vi "sendScript.vi"(8 "error in (no error)":errorcluster, 11 "K2602 in":refnum<class "K2602.lvclass">) -> (0 "error out":errorcluster, 3 "K2602 out":refnum<class "K2602.lvclass">)   [LabVIEW 2011, in "Hardware.lvlib" / "Channels.lvlib" / "K2602.lvclass"]
uses:
  K2602.lvclass
  K2602.lvclass/K2602.ctl
  <instrlib>/Keithley 2600 Series/Keithley 2600 Series.lvlib
panel:
  out "script":string
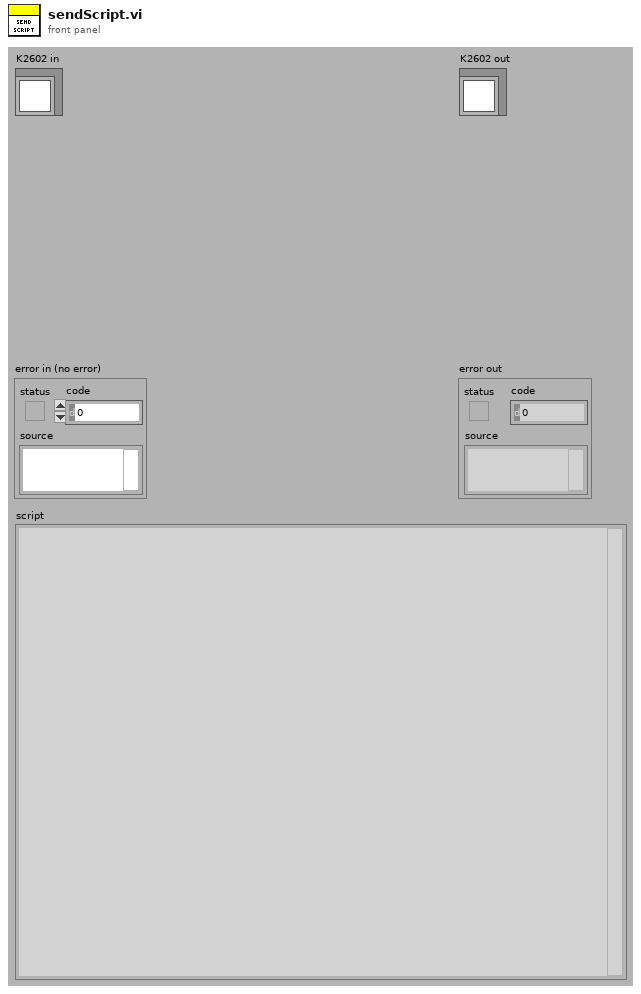
[diagram p1: front panel]
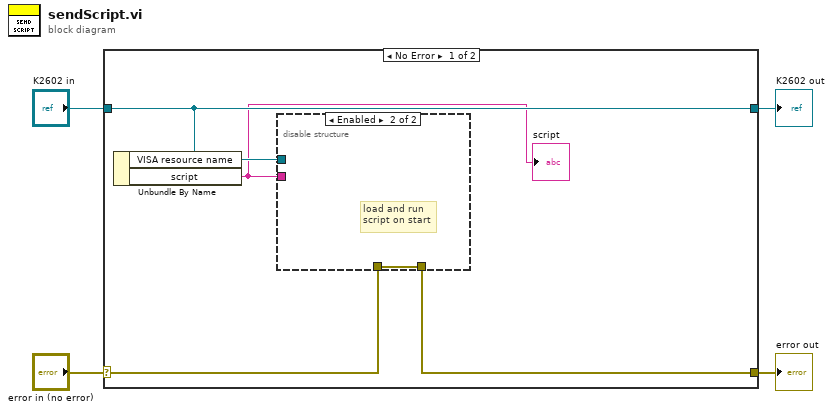
[diagram p0: block diagram]
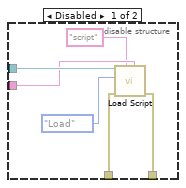
[diagram p2: hidden frame]
diagram:
  n1 = case shown="No Error" "error in (no error)" {
    selector: "error in (no error)" -> [w7 w18]
    tunnel: [w6 w18] -> w3
    tunnel: [w9 w17] -> w1
    tunnel: "K2602 in" -> [w9 w17]
    frame No Error {
      n2 = Unbundle By Name(w9) -> ("VISA resource name"=w8:refnum<visa-resource-name>, "script"=w5:string)
      "script" <- w5
      n3 = disable-structure shown="Enabled" {
        disable-tunnel: w8 -> [w15 _]
        disable-tunnel: w7 -> [w13 w16]
        disable-tunnel: [w12 w16] -> w6
        disable-tunnel: w5 -> [w11 _]
        frame Disabled {
          n4 = call <instrlib>:"Load Script.vi"("Script"=w11, "Script Name"="script", "error in"=w13, "Load Options (Load)"=enum16{"Load", "Load & Run"}."Load", "VISA resource name"=w15) -> ("error out"=w12:errorcluster)  [unwired: 4 in, 2 out]
        }
        frame Enabled {
          # "load and run\nscript on start"
        }
      }
    }
    frame Error {
    }
  }
  "error out" <- w3
  "K2602 out" <- w1
